vi "Filter_Evaluator.vi"(7 "Headers":string[](array[string])=["Packet Number", "Timestamp", "Source", "Destination", "Protocol", "Length", "Data"], 8 "Error":errorcluster, 9 "Comparators":T1(array[cluster]), 10 "Boolean Connectors":string[](array[string])=["AND", "OR"], 11 "Prefiltered Data":string[][](array[string])=array1500x7[10500 elements]) -> (0 "Error Out":errorcluster, 2 "Filtered Array":string[][](array[string]), 3 "Prefiltered Data":string[][](array[string]))   [LabVIEW 2025, in "Automotive Ethernet Bus Monitor UI.lvlib" / "Table_Filtering.lvlib"]
uses:
  Table_Filtering.lvlib
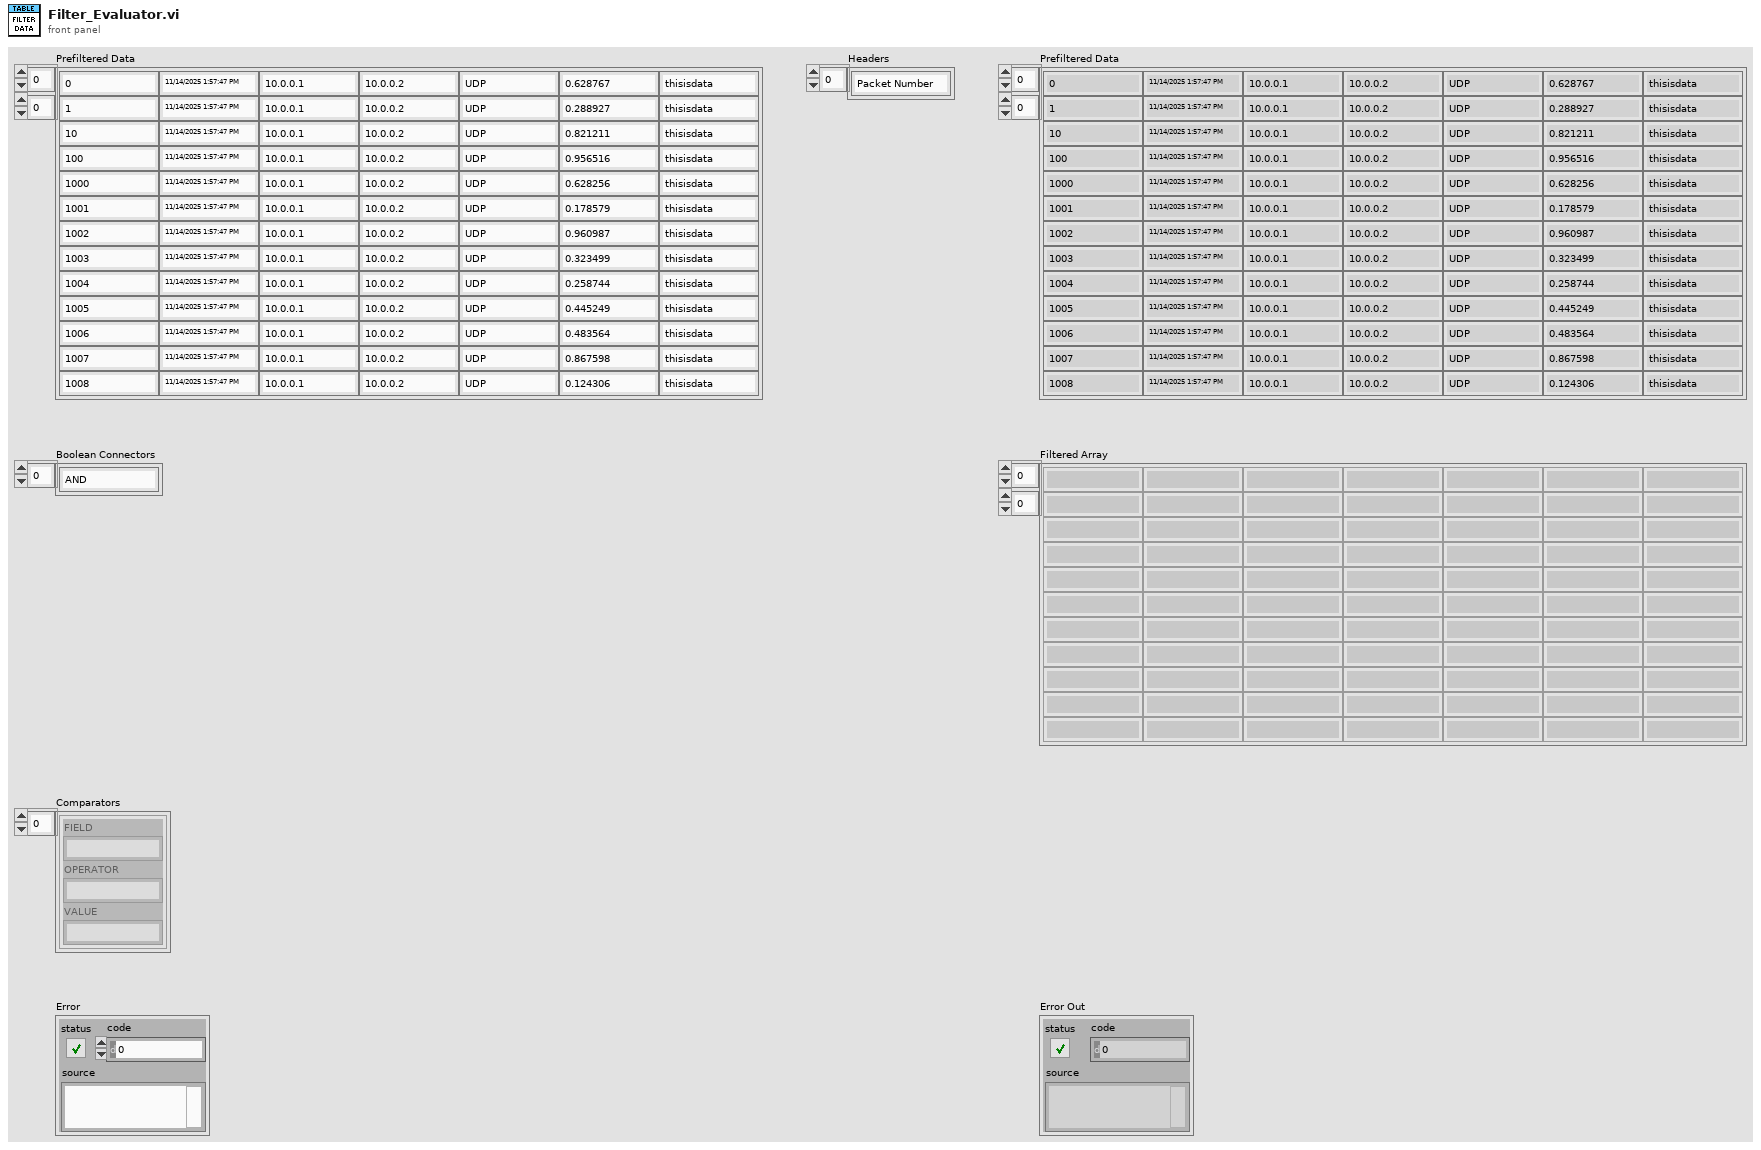
[diagram p1: front panel]
types:
  T1 = cluster{"FIELD":string, "OPERATOR":string, "VALUE":string}[]
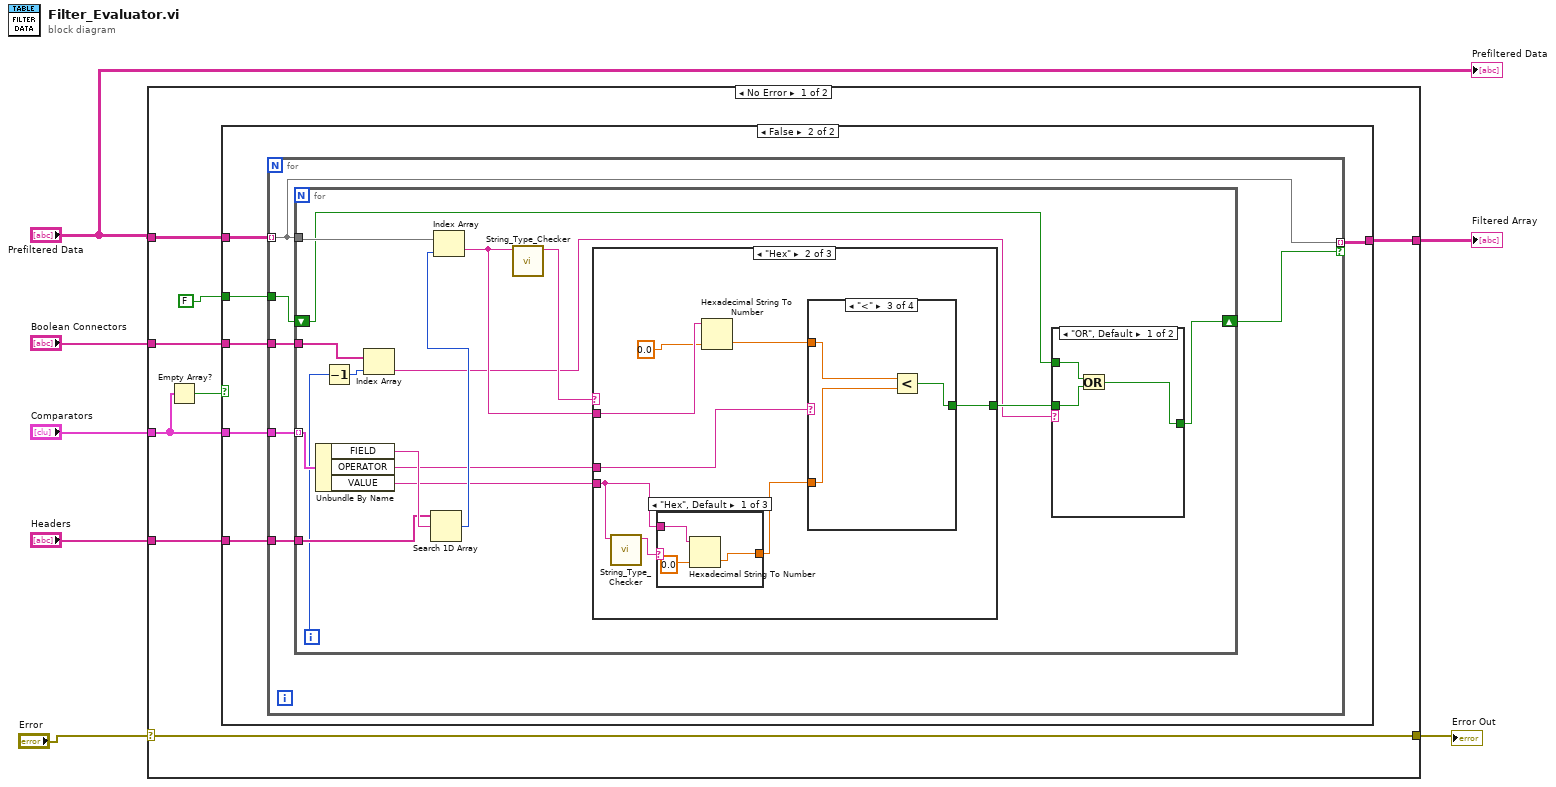
[diagram p0: block diagram]
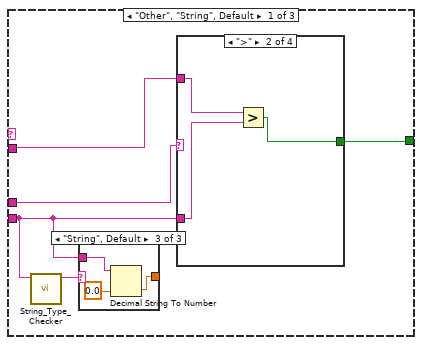
[diagram p3: hidden frame]
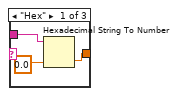
[diagram p4: hidden frame]
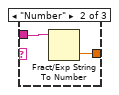
[diagram p5: hidden frame]
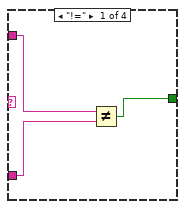
[diagram p6: hidden frame]
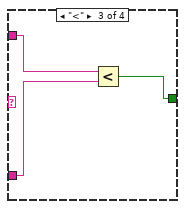
[diagram p7: hidden frame]
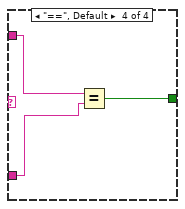
[diagram p8: hidden frame]
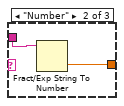
[diagram p9: hidden frame]
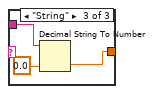
[diagram p10: hidden frame]
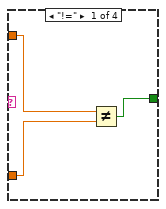
[diagram p11: hidden frame]
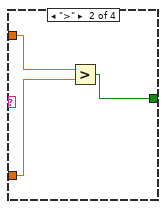
[diagram p12: hidden frame]
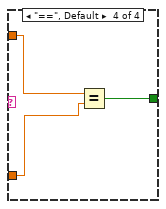
[diagram p13: hidden frame]
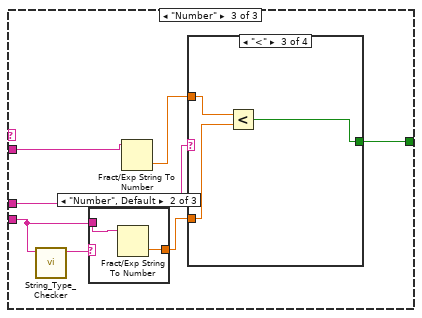
[diagram p14: hidden frame]
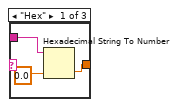
[diagram p15: hidden frame]
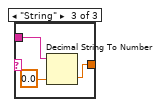
[diagram p16: hidden frame]
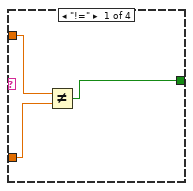
[diagram p17: hidden frame]
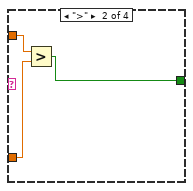
[diagram p18: hidden frame]
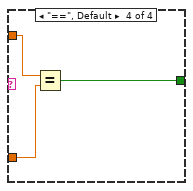
[diagram p19: hidden frame]
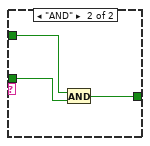
[diagram p20: hidden frame]
diagram:
  n1 = case shown="No Error" "Error" {
    selector: "Error" -> [w11 w131]
    tunnel: "Headers" -> [w15 _]
    tunnel: "Boolean Connectors" -> [w14 _]
    tunnel: "Comparators" -> [w8 _]
    tunnel: "Prefiltered Data" -> [w13 _]
    tunnel: [w12 _] -> w7
    tunnel: [w11 w131] -> w2
    frame No Error {
      n2 = Empty Array?(array=w8) -> (empty?=w9:bool)
      n3 = case shown="False" w9 {
        tunnel: w15 -> [_ w22]
        tunnel: FALSE -> [_ w21]
        tunnel: w14 -> [_ w20]
        tunnel: w8 -> [_ w19]
        tunnel: w13 -> [w16 w18]
        tunnel: [w16 w17] -> w12
        frame True {
        }
        frame False {
          n4 = for {
            tunnel: w22 -> [w28]
            tunnel: w19 -> [w27]
            tunnel: w18 -> [w23] mode=indexing
            tunnel: w21 -> [w26]
            tunnel: w20 -> [w25]
            tunnel: [w23] -> w17 mode=indexing if=w24
            n5 = for {
              tunnel: w28 -> [w41]
              tunnel: w27 -> [w44] mode=indexing
              tunnel: w23 -> [w43]
              shift-right: [w35] -> w24
              shift-left: w26 -> [w36]
              tunnel: w25 -> [w39]
              i -> [w37]
              n6 = Unbundle By Name(w44) -> ("FIELD"=w42:string, "OPERATOR"=w31:string, "VALUE"=w32:string)
              n7 = Decrement(x=w37) -> (x-1=w38:i32)
              n8 = Index Array(array=w39, index=w38) -> (element=w29:string)
              n9 = Search 1D Array(1D array=w41, element=w42) -> (index of element=w40:i32)  [unwired: 1 in]
              n10 = Index Array(array=w43, index=w40) -> (element=w33:string)
              n11 = call "String_Type_Checker.vi"("String"=w33) -> ("Type"=w34:string)  [unwired: 10 in]
              n12 = case shown="\"Hex\"" w34 {
                tunnel: w33 -> [w49 w77 w104]
                tunnel: w32 -> [w45 w71 w99]
                tunnel: w31 -> [w48 w75 w103]
                tunnel: [w47 w74 w101] -> w30
                frame "Other", "String", Default {
                  n13 = call "String_Type_Checker.vi"("String"=w45) -> ("Type"=w46:string)  [unwired: 10 in]
                  n14 = case shown="\"String\", Default" w46 {
                    tunnel: [w52 w54 w56] -> _
                    tunnel: w45 -> [w50 w53 w57]
                    frame "Hex" {
                      n15 = Hexadecimal String To Number(string=w50, default (0uL)=0.0) -> (number=w52:dbl)  [unwired: 1 in, 1 out]
                    }
                    frame "Number" {
                      n16 = Fract/Exp String To Number(string=w53) -> (number=w54:dbl)  [unwired: 3 in, 1 out]
                    }
                    frame "String", Default {
                      n17 = Decimal String To Number(string=w57, default (0L)=0.0) -> (number=w56:dbl)  [unwired: 1 in, 1 out]
                    }
                  }
                  n18 = case shown="\">\"" w48 {
                    tunnel: w49 -> [w59 w63 w66 w67]
                    tunnel: w45 -> [w58 w62 w65 w69]
                    tunnel: [w60 w61 w64 w68] -> w47
                    frame "!=" {
                      n19 = Not Equal?(x=w59, y=w58) -> (x != y?=w60:bool)
                    }
                    frame ">" {
                      n20 = Greater?(x=w63, y=w62) -> (0:w61:bool)
                    }
                    frame "<" {
                      n21 = Less?(x=w66, y=w65) -> (x < y?=w64:bool)
                    }
                    frame "==", Default {
                      n22 = Equal?(x=w67, y=w69) -> (x = y?=w68:bool)
                    }
                  }
                }
                frame "Hex" {
                  n23 = call "String_Type_Checker.vi"("String"=w71) -> ("Type"=w72:string)  [unwired: 10 in]
                  n24 = case shown="\"Hex\", Default" w72 {
                    tunnel: [w80 w82 w84] -> w73
                    tunnel: w71 -> [w78 w81 w85]
                    frame "Hex", Default {
                      n25 = Hexadecimal String To Number(string=w78, default (0uL)=0.0) -> (number=w80:dbl)  [unwired: 1 in, 1 out]
                    }
                    frame "Number" {
                      n26 = Fract/Exp String To Number(string=w81) -> (number=w82:dbl)  [unwired: 3 in, 1 out]
                    }
                    frame "String" {
                      n27 = Decimal String To Number(string=w85, default (0L)=0.0) -> (number=w84:dbl)  [unwired: 1 in, 1 out]
                    }
                  }
                  n28 = Hexadecimal String To Number(string=w77, default (0uL)=0.0) -> (number=w76:dbl)  [unwired: 1 in, 1 out]
                  n29 = case shown="\"<\"" w75 {
                    tunnel: w76 -> [w87 w91 w94 w95]
                    tunnel: w73 -> [w86 w90 w93 w97]
                    tunnel: [w88 w89 w92 w96] -> w74
                    frame "!=" {
                      n30 = Not Equal?(x=w87, y=w86) -> (x != y?=w88:bool)
                    }
                    frame ">" {
                      n31 = Greater?(x=w91, y=w90) -> (0:w89:bool)
                    }
                    frame "<" {
                      n32 = Less?(x=w94, y=w93) -> (x < y?=w92:bool)
                    }
                    frame "==", Default {
                      n33 = Equal?(x=w95, y=w97) -> (x = y?=w96:bool)
                    }
                  }
                }
                frame "Number" {
                  n34 = call "String_Type_Checker.vi"("String"=w99) -> ("Type"=w98:string)  [unwired: 10 in]
                  n35 = case shown="\"Number\", Default" w98 {
                    tunnel: [w107 w109 w111] -> w102
                    tunnel: w99 -> [w105 w108 w112]
                    frame "Hex" {
                      n36 = Hexadecimal String To Number(string=w105, default (0uL)=0.0) -> (number=w107:dbl)  [unwired: 1 in, 1 out]
                    }
                    frame "Number", Default {
                      n37 = Fract/Exp String To Number(string=w108) -> (number=w109:dbl)  [unwired: 3 in, 1 out]
                    }
                    frame "String" {
                      n38 = Decimal String To Number(string=w112, default (0L)=0.0) -> (number=w111:dbl)  [unwired: 1 in, 1 out]
                    }
                  }
                  n39 = Fract/Exp String To Number(string=w104) -> (number=w100:dbl)  [unwired: 3 in, 1 out]
                  n40 = case shown="\"<\"" w103 {
                    tunnel: w102 -> [w114 w118 w121 w124]
                    tunnel: [w115 w117 w120 w123] -> w101
                    tunnel: w100 -> [w113 w116 w119 w122]
                    frame "!=" {
                      n41 = Not Equal?(x=w113, y=w114) -> (x != y?=w115:bool)
                    }
                    frame ">" {
                      n42 = Greater?(x=w116, y=w118) -> (0:w117:bool)
                    }
                    frame "<" {
                      n43 = Less?(x=w119, y=w121) -> (x < y?=w120:bool)
                    }
                    frame "==", Default {
                      n44 = Equal?(x=w122, y=w124) -> (x = y?=w123:bool)
                    }
                  }
                }
              }
              n45 = case shown="\"OR\", Default" w29 {
                tunnel: w36 -> [w126 w130]
                tunnel: [w127 w129] -> w35
                tunnel: w30 -> [w125 w128]
                frame "OR", Default {
                  n46 = Or(x=w126, y=w125) -> (x .or. y?=w127:bool)
                }
                frame "AND" {
                  n47 = And(x=w130, y=w128) -> (x .and. y?=w129:bool)
                }
              }
            }
          }
        }
      }
    }
    frame Error {
    }
  }
  "Filtered Array" <- w7
  "Error Out" <- w2
  "Prefiltered Data" <- "Prefiltered Data"
